vi "Error Cluster From Code.vi"(5 "show call chain? (True)":bool=TRUE, 6 "error in (no error)":errorcluster, 7 "Call Depth":i32, 8 "error message (\"\")":string, 9 "error code (402840+)":i32=402842) -> (0 "error out":errorcluster)   [LabVIEW 2019, in "JSONtext.lvlib"]
doc: "Converts an error or warning code to an error cluster. This VI is useful when you receive a return value from a shared library call or when you return user-defined error codes."
uses:
  JSONtext.lvlib
panel:
  in  "call chain header":string="\n<b>Complete call chain:</b>"
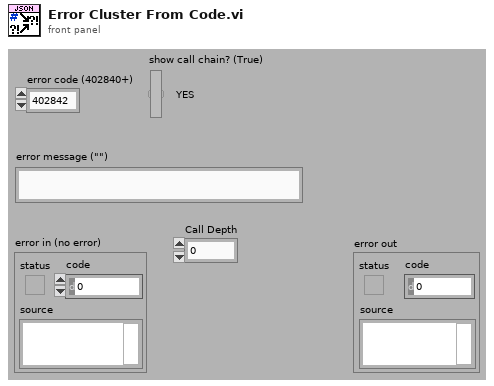
[diagram p1: front panel]
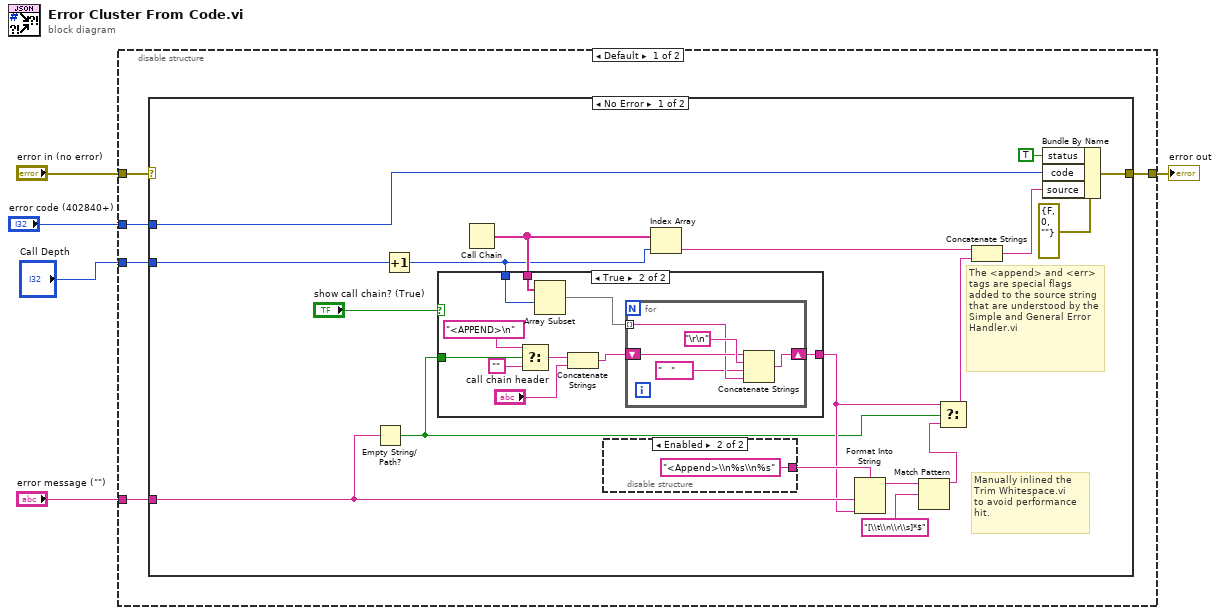
[diagram p0: block diagram]
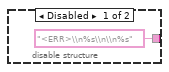
[diagram p2: hidden frame]
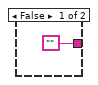
[diagram p3: hidden frame]
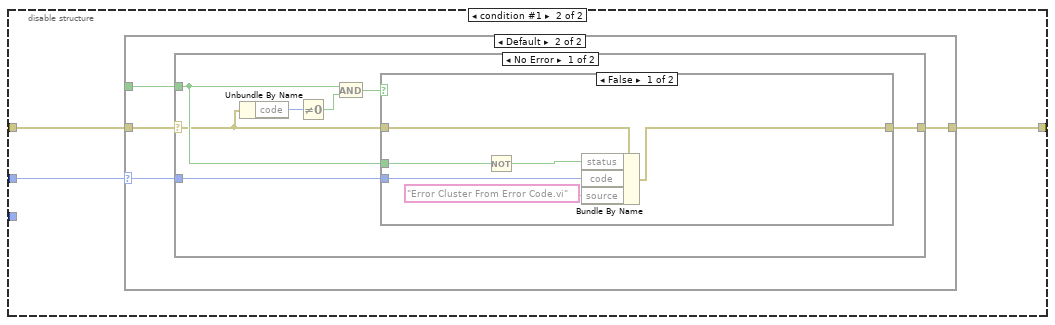
[diagram p5: hidden frame]
diagram:
  n1 = disable-structure shown="Default" {
    disable-tunnel: [w10 w50] -> w5
    disable-tunnel: "error in (no error)" -> [w9 w51]
    disable-tunnel: "error code (402840+)" -> [w8 w49]
    disable-tunnel: "error message (\"\")" -> [w7 _]
    disable-tunnel: "Call Depth" -> [w6 _]
    frame condition #0 (active) {
      n2 = case shown="No Error" w9 {
        selector: w9 -> [_ w47]
        tunnel: [w28 w47] -> w10
        tunnel: w8 -> [w27 _]
        tunnel: w7 -> [w26 _]
        tunnel: w6 -> [w25 _]
        frame No Error {
          # "Manually inlined the\nTrim Whitespace.vi\nto avoid performance\nhit."
          # "The <append> and <err> tags are special flags added to the source string that are understood by the Simple and General Error Handler.vi"
          n3 = Empty String/Path?(string/path=w26) -> (empty?=w17:bool)
          n4 = Increment(x=w25) -> (x+1=w12:i32)
          n5 = Call Chain() -> (call chain=w22:string[])
          n6 = case shown="True" "show call chain? (True)" {
            tunnel: ["" w41] -> w19
            tunnel: w22 -> [_ w40]
            tunnel: w17 -> [_ w36]
            tunnel: w12 -> [_ w32]
            frame False {
            }
            frame True {
              n7 = Select(t="<APPEND>\n", s=w36, f="") -> (s? t:f=w33:string)
              n8 = Array Subset(array=w40, index=w32) -> (w39:string[])  [unwired: 1 in]
              n9 = Concatenate Strings(w33, "call chain header") -> (w37:string)
              n10 = for {
                tunnel: w39 -> [w43] mode=indexing
                shift-right: [w46] -> w41
                shift-left: w37 -> [w44]
                n11 = Concatenate Strings(w44, "\r\n", "   ", w43) -> (w46:string)
              }
            }
          }
          n12 = disable-structure shown="Enabled" {
            disable-tunnel: ["<ERR>\\n%s\\n\\n%s" ("format string") "<Append>\\n%s\\n%s" ("format string")] -> w20
            frame Disabled {
            }
            frame Enabled {
            }
          }
          n13 = Index Array(array=w22, index=w12) -> (element=w13:string)
          n14 = Format Into String(format string=w20, w26, w19) -> (resulting string=w15:string)  [unwired: 2 in, 1 out]
          n15 = Match Pattern(string=w15, regular expression="[\\t\\n\\r\\s]*$") -> (before substring=w14:string)  [unwired: 1 in, 3 out]
          n16 = Select(t=w19, s=w17, f=w14) -> (s? t:f=w18:string)
          n17 = Concatenate Strings(w13, w18) -> (w23:string)
          n18 = Bundle By Name(cluster=errorcluster {"status"=FALSE, "code"=0, "source"=""} ("error out"), "status"=TRUE, "code"=w27, "source"=w23) -> (w28:errorcluster)
        }
        frame Error {
          # "An error in trumps any error code input."
        }
      }
    }
    frame condition #1 {
      n19 = case shown="Default" w49 {
        selector: w49 -> [_ w54]
        tunnel: w51 -> [w52 w56]
        tunnel: [w52 w55] -> w50
        tunnel: [_ w53] -> w48
        frame 0 {
          # "If the error code in equals zero, then propagate the error in cluster regardless of its value."
        }
        frame Default {
          n20 = case shown="No Error" w56 {
            selector: w56 -> [w58 w71]
            tunnel: [w62 w71] -> w55
            tunnel: w54 -> [w63 _]
            tunnel: w53 -> [w59 _]
            frame No Error {
              n21 = Unbundle By Name(w58) -> ("code"=w61:i32)
              n22 = Not Equal To 0?(x=w61) -> (x != 0?=w60:bool)
              n23 = And(x=w59, y=w60) -> (x .and. y?=w57:bool)
              n24 = case shown="False" w57 {
                tunnel: w63 -> [w69 _]
                tunnel: [w66 w70] -> w62
                tunnel: w59 -> [w65 _]
                tunnel: w58 -> [w64 w70]
                frame False {
                  n25 = Not(x=w65) -> (.not. x?=w68:bool)
                  n26 = Bundle By Name(cluster=w64, "status"=w68, "code"=w69, "source"="Error Cluster From Error Code.vi") -> (w66:errorcluster)
                }
                frame True {
                  # "If the error code input is setting a warning, and a warning is already set on the wire, then we\ngo with the one already on the wire."
                }
              }
            }
            frame Error {
              # "An error in trumps any error code input."
            }
          }
        }
      }
    }
  }
  "error out" <- w5
